vi "_050.vi"() -> ()   [LabVIEW 2024]
panel:
  out "You order will preparing":dbl
  in  "Pay Bill & Comform":bool
  out "Discount":string
  out "Total Bill":dbl
  in  "Item#1 5":bool
  in  "Quantity 5":dbl=1.0 min=1.0 max=10.0 step=1.0
  out "Price 5":dbl
  in  "Item#1 4":bool
  in  "Quantity 4":dbl=1.0 min=1.0 max=10.0 step=1.0
  out "Price 4":dbl
  in  "Item#1 3":bool
  in  "Quantity 3":dbl=1.0 min=1.0 max=10.0 step=1.0
  out "Price 3":dbl
  in  "Item#1 2":bool
  in  "Quantity 2":dbl=1.0 min=1.0 max=10.0 step=1.0
  out "Price 2":dbl
  out "Price":dbl
  in  "Quantity":dbl=1.0 min=1.0 max=10.0 step=1.0
  in  "Item#1":bool
  # "Food Ordering System :"
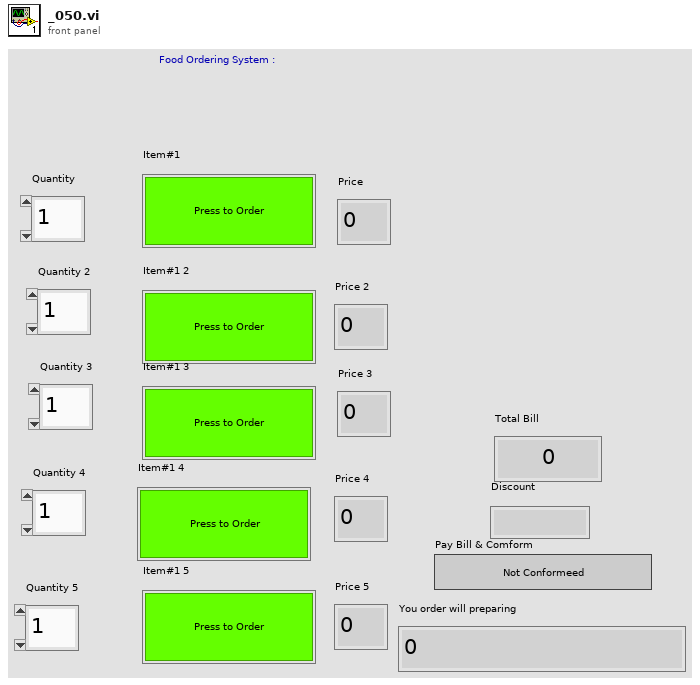
[diagram p1: front panel]
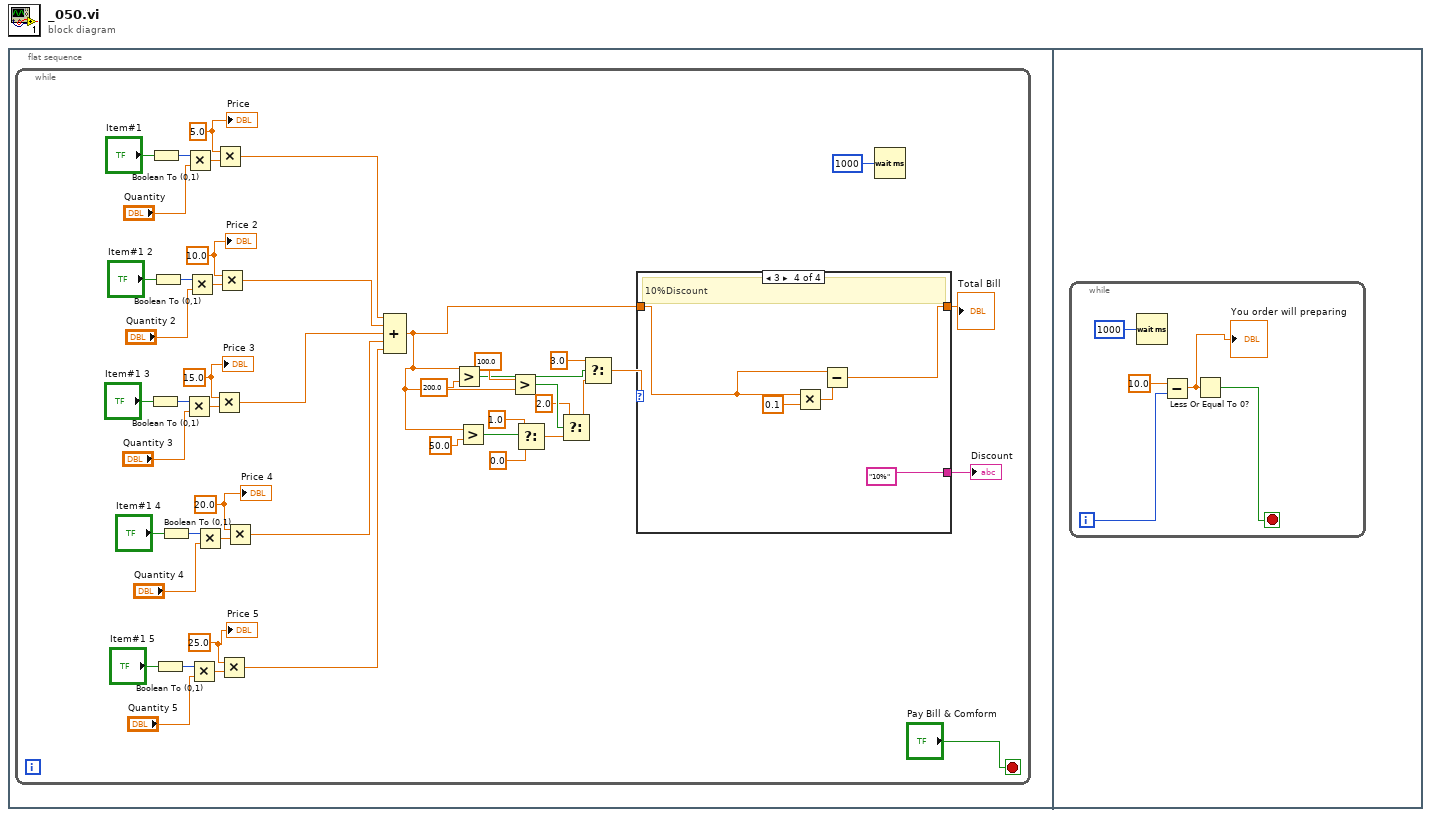
[diagram p0: block diagram]
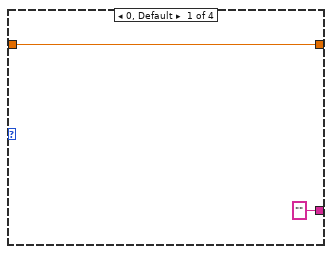
[diagram p2: hidden frame]
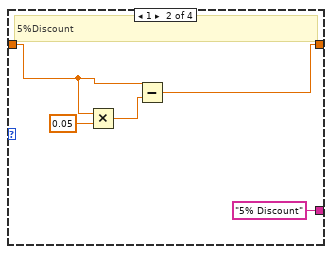
[diagram p3: hidden frame]
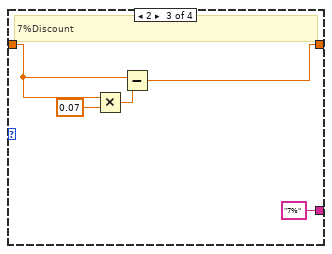
[diagram p4: hidden frame]
diagram:
  n1 = flat-sequence {
    frame #0 {
      n2 = while {
        stop <- "Pay Bill & Comform" stop-if-true
        w28 = 25.0 ("x")
        w29 = 20.0 ("x")
        w38 = 15.0 ("x")
        w43 = 10.0 ("x")
        w44 = 5.0 ("x")
        n3 = Boolean To (0,1)(Boolean="Item#1 3") -> (0, 1=w36:i16)
        n4 = Boolean To (0,1)(Boolean="Item#1") -> (0, 1=w46:i16)
        n5 = Boolean To (0,1)(Boolean="Item#1 2") -> (0, 1=w41:i16)
        n6 = Boolean To (0,1)(Boolean="Item#1 5") -> (0, 1=w26:i16)
        n7 = Boolean To (0,1)(Boolean="Item#1 4") -> (0, 1=w31:i16)
        n8 = Multiply(x=w36, y="Quantity 3") -> (x*y=w37:dbl)
        n9 = Multiply(x=w46, y="Quantity") -> (x*y=w45:dbl)
        n10 = Multiply(x=w41, y="Quantity 2") -> (x*y=w42:dbl)
        n11 = Multiply(x=w26, y="Quantity 5") -> (x*y=w27:dbl)
        n12 = Multiply(x=w31, y="Quantity 4") -> (x*y=w30:dbl)
        n13 = Multiply(x=w38, y=w37) -> (x*y=w21:dbl)
        n14 = Multiply(x=w44, y=w45) -> (x*y=w23:dbl)
        n15 = Multiply(x=w43, y=w42) -> (x*y=w22:dbl)
        n16 = Multiply(x=w28, y=w27) -> (x*y=w19:dbl)
        n17 = Multiply(x=w29, y=w30) -> (x*y=w20:dbl)
        n18 = Compound Arithmetic op=ADD(w23, w22, w21, w20, w19) -> (w6:dbl)
        n19 = Greater?(x=w6, y=200.0) -> (0:w8:bool)
        n20 = Greater?(x=w6, y=50.0) -> (0:w17:bool)
        n21 = Greater?(x=100.0 ("t"), y=w6) -> (0:w7:bool)
        n22 = Select(t=1.0, s=w17, f=0.0) -> (s? t:f=w5:dbl)
        n23 = Select(t=2.0, s=w7, f=w5) -> (s? t:f=w3:dbl)
        n24 = Select(t=3.0, s=w8, f=w3) -> (s? t:f=w1:dbl)
        n25 = case shown="3" w1 {
          tunnel: [w50 w52 w57 w63] -> w14
          tunnel: w6 -> [w50 w53 w58 w61]
          tunnel: ["" ("String") "5% Discount" ("String") "7%" ("String") "10%"] -> w13
          frame 0, Default {
          }
          frame 1 {
            # "5%Discount"
            n26 = Multiply(x=w53, y=0.05) -> (x*y=w51:dbl)
            n27 = Subtract(x=w53, y=w51) -> (x-y=w52:dbl)
          }
          frame 2 {
            # "7%Discount"
            n28 = Multiply(x=w58, y=0.07) -> (x*y=w59:dbl)
            n29 = Subtract(x=w58, y=w59) -> (x-y=w57:dbl)
          }
          frame 3 {
            # "10%Discount"
            n30 = Multiply(x=w61, y=0.1) -> (x*y=w65:dbl)
            n31 = Subtract(x=w61, y=w65) -> (x-y=w63:dbl)
          }
        }
        "Total Bill" <- w14
        "Discount" <- w13
        n32 = Wait (ms)(milliseconds to wait=u32 1000 ("millisecond timer value")) -> ()  [unwired: 1 out]
        "Price" <- w44
        "Price 2" <- w43
        "Price 3" <- w38
        "Price 4" <- w29
        "Price 5" <- w28
      }
    }
    frame #1 {
      n33 = while {
        i -> [w69]
        stop <- w68 stop-if-true
        n34 = Wait (ms)(milliseconds to wait=u32 1000 ("millisecond timer value")) -> ()  [unwired: 1 out]
        n35 = Subtract(x=10.0, y=w69) -> (x-y=w67:dbl)
        "You order will preparing" <- w67
        n36 = Less Or Equal To 0?(x=w67) -> (x <= 0?=w68:bool)
      }
    }
  }
